vi "GEN40-38-LAN Verify Current Setting.vi"(8 "error in (no error)":errorcluster, 11 "GEN40-38-LAN in":refnum<class "GEN40-38-LAN.lvclass">) -> (0 "error out":errorcluster, 3 "GEN40-38-LAN out":refnum<class "GEN40-38-LAN.lvclass">)   [LabVIEW 2018, in "GEN40-38-LAN.lvlib" / "GEN40-38-LAN.lvclass"]
uses:
  GEN40-38-LAN.lvclass
  GEN40-38-LAN.lvclass/GEN40-38-LAN.ctl
  PPLs/Power Supply/Parent/Power_Supply.lvlibp/Power Supply.lvclass
  C:/Projects/LabVIEW/PPLs/Power Supply/Parent/Power_Supply.lvlibp/Power Supply.lvclass
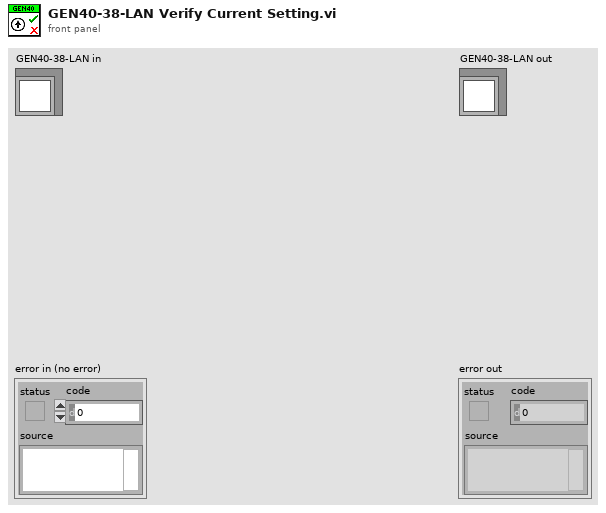
[diagram p1: front panel]
types:
  T1 = typedef "Power_Supply.lvlibp/Supply Settings.ctl" = cluster{"Voltage":dbl, "Current":dbl, "Output":bool}
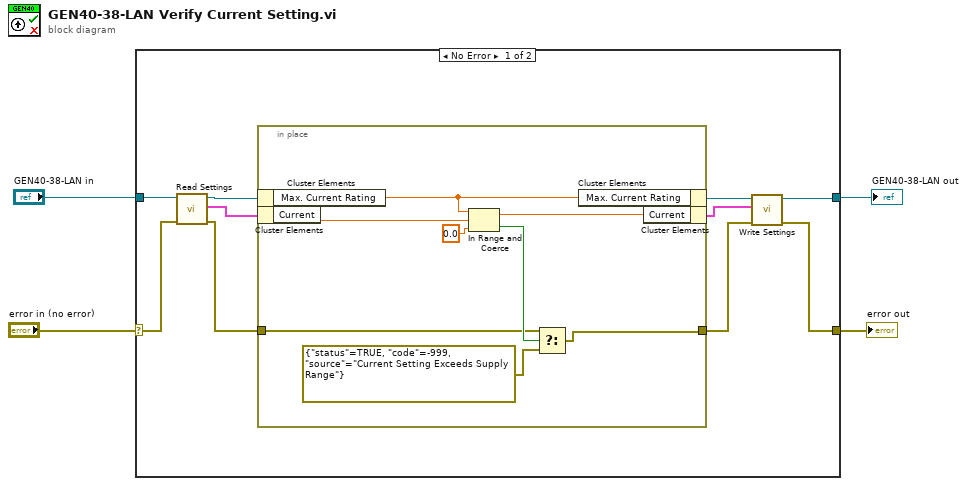
[diagram p0: block diagram]
diagram:
  n1 = case shown="No Error" "error in (no error)" {
    selector: "error in (no error)" -> [w13 w24]
    tunnel: [w6 w24] -> w3
    tunnel: [w5 w23] -> w1
    tunnel: "GEN40-38-LAN in" -> [w14 w23]
    frame No Error {
      n2 = call "Read Settings.vi"("error in (no error)"=w13, "Power Supply in"=w14) -> ("error out"=w10:errorcluster, "Settings"=w11:T1, "Power Supply out"=w12:refnum<class "GEN40-38-LAN.lvclass">)  [unwired: 7 in]
      n3 = in-place {
        in-place-border: w10 -> [w17]
        in-place-border: [w16] -> w7
        n4 = in-place-cluster #1(w12) -> ("Max. Current Rating"=w22:dbl)
        n5 = in-place-cluster #2(w11) -> ("Current"=w21:dbl)
        n6 = In Range and Coerce(upper limit=w22, x=w21, lower limit=0.0) -> (coerced(x)=w19:dbl, In Range?=w18:bool)
        n7 = Select(t=w17, s=w18, f=errorcluster {"status"=TRUE, "code"=-999, "source"="Current Setting Exceeds Supply Range"}) -> (s? t:f=w16:errorcluster)
        n8 = in-place-cluster #1("Max. Current Rating"=w22) -> (w9:refnum<class "GEN40-38-LAN.lvclass">)
        n9 = in-place-cluster #2("Current"=w19) -> (w8:T1)
      }
      n10 = call "Write Settings.vi"("error in (no error)"=w7, "Settings"=w8, "Power Supply in"=w9) -> ("error out"=w6:errorcluster, "Power Supply out"=w5:refnum<class "GEN40-38-LAN.lvclass">)  [unwired: 7 in]
    }
    frame Error {
    }
  }
  "error out" <- w3
  "GEN40-38-LAN out" <- w1
